vi "RT Comm Refs.vi"() -> ()   [LabVIEW 2014]
uses:
  Controls/RT Stream Data.ctl
panel:
  in  "reader endpoint":refnum<k21>
  in  "writer endpoint":refnum<k21>
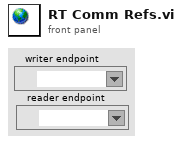
[diagram p1: front panel]
diagram:
